vi "Receive Event.vi"(8 "Error In":errorcluster, 9 "Event Data":refnum<class "Event Data.lvclass">, 10 "Event Name":string, 11 "Example logger In":refnum<class "Example logger.lvclass">) -> (0 "Error Out":errorcluster, 3 "Example logger Out":refnum<class "Example logger.lvclass">)   [LabVIEW 2020, in "Example logger.lvlib" / "Example logger.lvclass"]
uses:
  Example logger.lvclass
  Source/Template Source/Event Data/Event Data.lvclass
  Doublo Array/Doublo Array.lvclass
  Doublo Array/Doublo Array.lvclass/Doublo Array.ctl
  Timestamp/Timestamp.lvclass
  Timestamp/Timestamp.lvclass/Timestamp.ctl
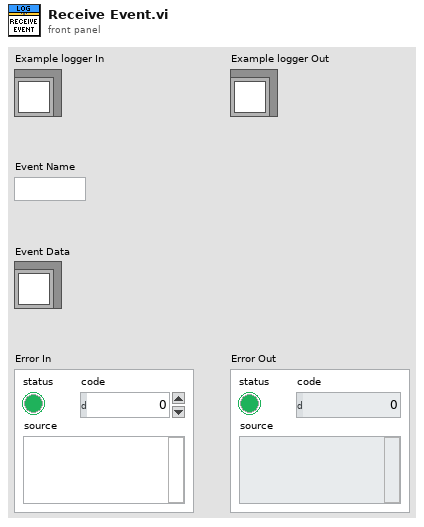
[diagram p1: front panel]
types:
  T1 = enum16{"open", "replace", "create", "open or create", "replace or create", "replace or create with confirmation"}
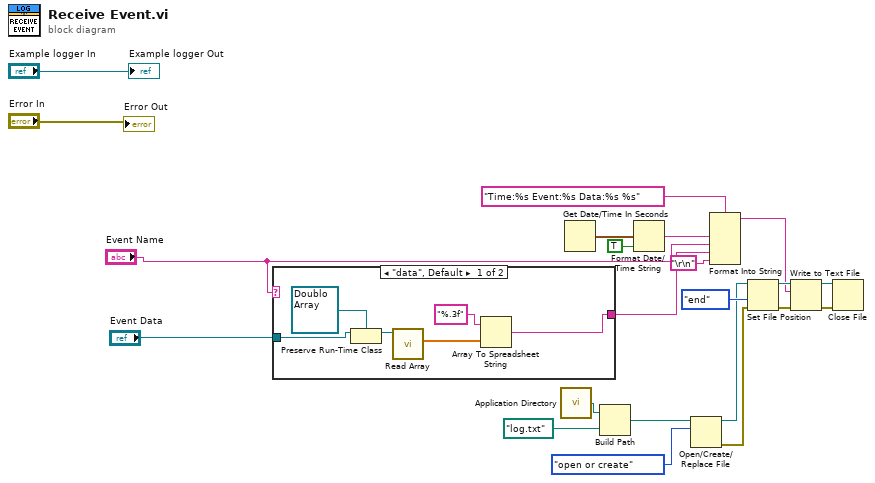
[diagram p0: block diagram]
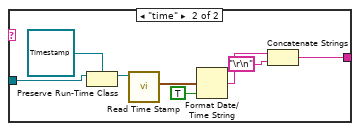
[diagram p2: hidden frame]
diagram:
  n1 = case shown="\"data\", Default" "Event Name" {
    tunnel: "Event Data" -> [w28 w36]
    tunnel: [w23 w29] -> w9
    frame "data", Default {
      n2 = Preserve Run-Time Class(object in=w28, 2:refnum<class "Doublo Array.lvclass"> refnum ("Example Source.lvlib:Doublo Array.lvclass")) -> (object out=w26:refnum<class "Doublo Array.lvclass">)  [unwired: 1 in, 1 out]
      n3 = call "Read Array.vi"("Doublo Array in"=w26) -> ("Array"=w25:dbl[])  [unwired: 8 in, 2 out]
      n4 = Array To Spreadsheet String(array=w25, 3:"%.3f" ("format string")) -> (spreadsheet string=w23:string)  [unwired: 1 in]
    }
    frame "time" {
      n5 = Preserve Run-Time Class(object in=w36, 2:refnum<class "Timestamp.lvclass"> refnum ("Example Source.lvlib:time.lvclass")) -> (object out=w34:refnum<class "Timestamp.lvclass">)  [unwired: 1 in, 1 out]
      n6 = call "Read Time Stamp.vi"("time in"=w34) -> ("Time Stamp"=w33:timestamp)  [unwired: 8 in, 2 out]
      n7 = Format Date/Time String(seconds (now)=w33, UTC format=TRUE) -> (date/time string=w31:string)  [unwired: 1 in]
      n8 = Concatenate Strings(w31, "\r\n") -> (w29:string)
    }
  }
  n9 = call <vilib>:"Application Directory.vi"() -> ("Application Directory"=w21:path)
  n10 = Get Date/Time In Seconds() -> (seconds since 1Jan1904=w4:timestamp)
  n11 = Build Path(base path=w21, name or relative path=path "log.txt") -> (appended path=w19:path)
  n12 = Format Date/Time String(seconds (now)=w4, UTC format=TRUE) -> (date/time string=w7:string)  [unwired: 1 in]
  n13 = Open/Create/Replace File(file path (use dialog)=w19, operation (0:open)=T1."open or create") -> (refnum out=w14:refnum<file>, error out=w12:errorcluster)  [unwired: 4 in, 1 out]
  n14 = Format Into String(format string="Time:%s Event:%s Data:%s %s", w7, "Event Name", w9, "\r\n") -> (resulting string=w6:string)  [unwired: 2 in, 1 out]
  n15 = Set File Position(refnum=w14, from (0:start)=enum16{"start", "end", "current"}."end", error in=w12) -> (refnum out=w13:refnum<file>, error out=w11:errorcluster)  [unwired: 1 in]
  n16 = Write to Text File(file (use dialog)=w13, text=w6, error in=w11) -> (refnum out=w18:refnum<file>, error out=w17:errorcluster)  [unwired: 1 in, 1 out]
  n17 = Close File(refnum=w18, error in=w17) -> ()  [unwired: 2 out]
  "Example logger Out" <- "Example logger In"
  "Error Out" <- "Error In"
